vi "Stop_Data_Loop.vi"() -> ()   [LabVIEW 2012]
panel:
  out "Stop data loop":bool
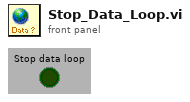
[diagram p1: front panel]
diagram:
